vi "PropertyNodes.vi"() -> ()   [LabVIEW 2018]
panel:
  in  "?":bool
  out "Boolean":bool
  # "Blue"
  # "Green"
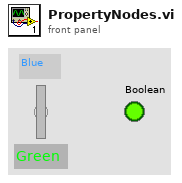
[diagram p1: front panel]
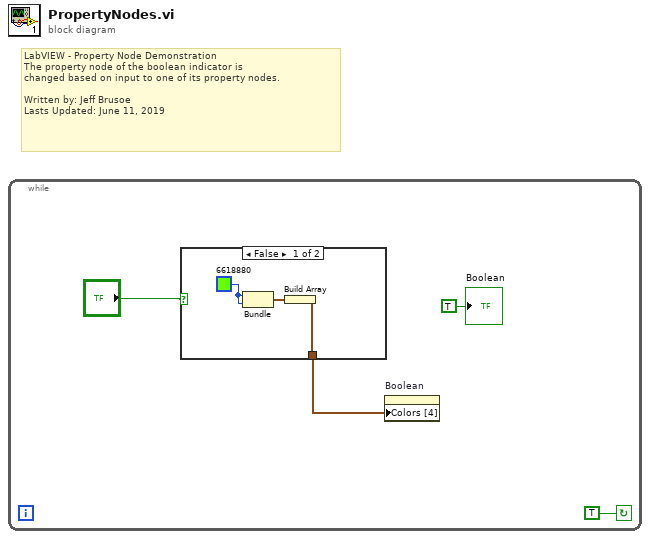
[diagram p0: block diagram]
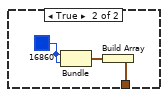
[diagram p2: hidden frame]
diagram:
  # "LabVIEW - Property Node Demonstration\nThe property node of the boolean indicator is\nchanged based on input to one of its property nodes.\n\nWritten by: Jeff Brusoe\nLasts Updated: June 11, 2019"
  n1 = while {
    stop <- TRUE continue-if-true
    n2 = case shown="False" "?" {
      tunnel: [w5 w8] -> w1
      frame False {
        w6 = u32 6618880
        n3 = Bundle(w6, w6) -> (w7:cluster{u32, u32})  [unwired: 1 in]
        n4 = Build Array(w7) -> (w5:cluster{u32, u32}[])
      }
      frame True {
        w9 = u32 16860
        n5 = Bundle(w9, w9) -> (w10:cluster{u32, u32})  [unwired: 1 in]
        n6 = Build Array(w10) -> (w8:cluster{u32, u32}[])
      }
    }
    n7 = property on="Boolean" class="Bool (strict)"("Colors [4]"=w1) -> ()  [unwired: 2 in, 2 out]
    "Boolean" <- TRUE ("Boolean")
  }
